vi "中间变量.vi"() -> ()   [LabVIEW 2016, in "PLC.lvlib"]
uses:
  PLC.lvlib
  <vilib>/Plasmionique/MB Master/MB_Master_Serial/MB_Master_Serial.lvclass
panel:
  in  "MB_Serial session":refnum<class "MB_Master_Serial.lvclass">
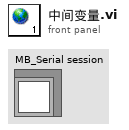
[diagram p1: front panel]
diagram:
